vi "SIM Integrator collector (for core) (vector).vi"(8 "DNL_Simulation CallChain":string, 9 "input":dbl[](array[numeric]), 10 "width":i32, 11 "Simulation data":T1={"continuous integrator"=enum."RK 1 (Euler)", "initial time"=0.0, "final time"=0.0, "step size"=0.0, "proposed step size"=0.0, "max step size"=0.0, "min step size"=0.0, "discrete time step"=0.0, "max step ratio"=0.0, "Diag Eval Stage"=enum."Init", "Substep Index"=0, "Timestep Index"=0.0, "simulation time"=0.0, "current timestep base"=0.0, "proposed step time"=0.0, "absolute tolerance"=0.0, "relative tolerance"=0.0, "step accepted?"=FALSE, "step complete?"=FALSE, "Halt?"=FALSE, "reset integrator?"=FALSE, "machine epsilon"=0.0, "min float"=0.0, "error"={"status"=FALSE, "code"=0, "source"=""}, "Method Order"=0, "Finished Late [i-1]"=FALSE, "Discrete step?"=FALSE, "NaN and Inf check?"=FALSE, "Final Timestep Index"=0.0, "(maj+disc)or(init)?"=FALSE, "Full Solver Reset"=TRUE, "Execution Mode"=enum."Simulate to Completion", "check vector sizes?"=FALSE, "solver handles zc?"=FALSE, "Simulation Registry"={"Current Idx"=0, "Node Tags"=[], "Node Headers"=[], "Node Data"=[], "Cont State data"={"inputs"=[], "outputs"=[], "reset"=[], "lower limits"=[], "upper limits"=[], "limit types"=[], "reset types"=[], "initial conditions"=[], "reset I.C."=[], "limited?"=[], "State Names"=[]}, "DiscreteInfo"={"tick period (sec)"=0.0, "time (ticks)"=0, "fire?"=[], "registry"={"period (sec)"=[], "skew (sec)"=[], "period (tick)"=[], "skew (tick)"=[]}, "discrete \nblocks?"=FALSE, "steps per tick"=0.0, "steps to tick"=0.0, "discrete \ntick?"=FALSE}, "Disc State data"={"Disc States"=[], "State Names"=[]}, "Registry Error"={"Error Block ID"=0, "code"=0}, "ZC Indices"=[]}, "variable step solver?"=FALSE, "First Substep?"=FALSE, "Continuous States?"=FALSE} {"min float" format="%.1e"; "proposed step size" format="%.1e"; "proposed step time" format="%.1e"; "max step ratio" format="%.1e"; "min step size" format="%.1e"; "machine epsilon" format="%.1e"; "discrete time step" format="%.1e"; "max step size" format="%.1e"; "current timestep base" format="%.1e"; "final time" format="%.1e"; "simulation time" format="%.1e"; "relative tolerance" format="%.1e"; "absolute tolerance" format="%.1e"; "Substep Index" format="%.1e"; "step size" format="%.1e"; "initial time" format="%.1e"}) -> (3 "Simulation data out":T1={"continuous integrator"=enum."RK 1 (Euler)", "initial time"=0.0, "final time"=0.0, "step size"=0.0, "proposed step size"=0.0, "max step size"=0.0, "min step size"=0.0, "discrete time step"=0.0, "max step ratio"=0.0, "Diag Eval Stage"=enum."Init", "Substep Index"=0, "Timestep Index"=0.0, "simulation time"=0.0, "current timestep base"=0.0, "proposed step time"=0.0, "absolute tolerance"=0.0, "relative tolerance"=0.0, "step accepted?"=FALSE, "step complete?"=FALSE, "Halt?"=FALSE, "reset integrator?"=FALSE, "machine epsilon"=0.0, "min float"=0.0, "error"={"status"=FALSE, "code"=0, "source"=""}, "Method Order"=0, "Finished Late [i-1]"=FALSE, "Discrete step?"=FALSE, "NaN and Inf check?"=FALSE, "Final Timestep Index"=0.0, "(maj+disc)or(init)?"=FALSE, "Full Solver Reset"=TRUE, "Execution Mode"=enum."Simulate to Completion", "check vector sizes?"=FALSE, "solver handles zc?"=FALSE, "Simulation Registry"={"Current Idx"=0, "Node Tags"=[], "Node Headers"=[], "Node Data"=[], "Cont State data"={"inputs"=[], "outputs"=[], "reset"=[], "lower limits"=[], "upper limits"=[], "limit types"=[], "reset types"=[], "initial conditions"=[], "reset I.C."=[], "limited?"=[], "State Names"=[]}, "DiscreteInfo"={"tick period (sec)"=0.0, "time (ticks)"=0, "fire?"=[], "registry"={"period (sec)"=[], "skew (sec)"=[], "period (tick)"=[], "skew (tick)"=[]}, "discrete \nblocks?"=FALSE, "steps per tick"=0.0, "steps to tick"=0.0, "discrete \ntick?"=FALSE}, "Disc State data"={"Disc States"=[], "State Names"=[]}, "Registry Error"={"Error Block ID"=0, "code"=0}, "ZC Indices"=[]}, "variable step solver?"=FALSE, "First Substep?"=FALSE, "Continuous States?"=FALSE} {"min float" format="%.1e"; "proposed step size" format="%.1e"; "proposed step time" format="%.1e"; "max step ratio" format="%.1e"; "min step size" format="%.1e"; "machine epsilon" format="%.1e"; "discrete time step" format="%.1e"; "max step size" format="%.1e"; "current timestep base" format="%.1e"; "final time" format="%.1e"; "simulation time" format="%.1e"; "relative tolerance" format="%.1e"; "absolute tolerance" format="%.1e"; "Substep Index" format="%.1e"; "step size" format="%.1e"; "initial time" format="%.1e"})   [LabVIEW 2014]
uses:
  SIM simulation data.ctl
  SIM integration method.ctl
  SIM diagram eval stage.ctl
  SIMSCR Execution Mode.ctl
  SIM Simulation Registry.ctl
  SIM Registry Node Header.ctl
  SIM Registry Node Record.ctl
  SIM trigger type.ctl
  SIM solver state data.ctl
  SIM limit type.ctl
  SIM discrete data.ctl
  SIM Discrete state data.ctl
  SIM Simulation Registry Error.ctl
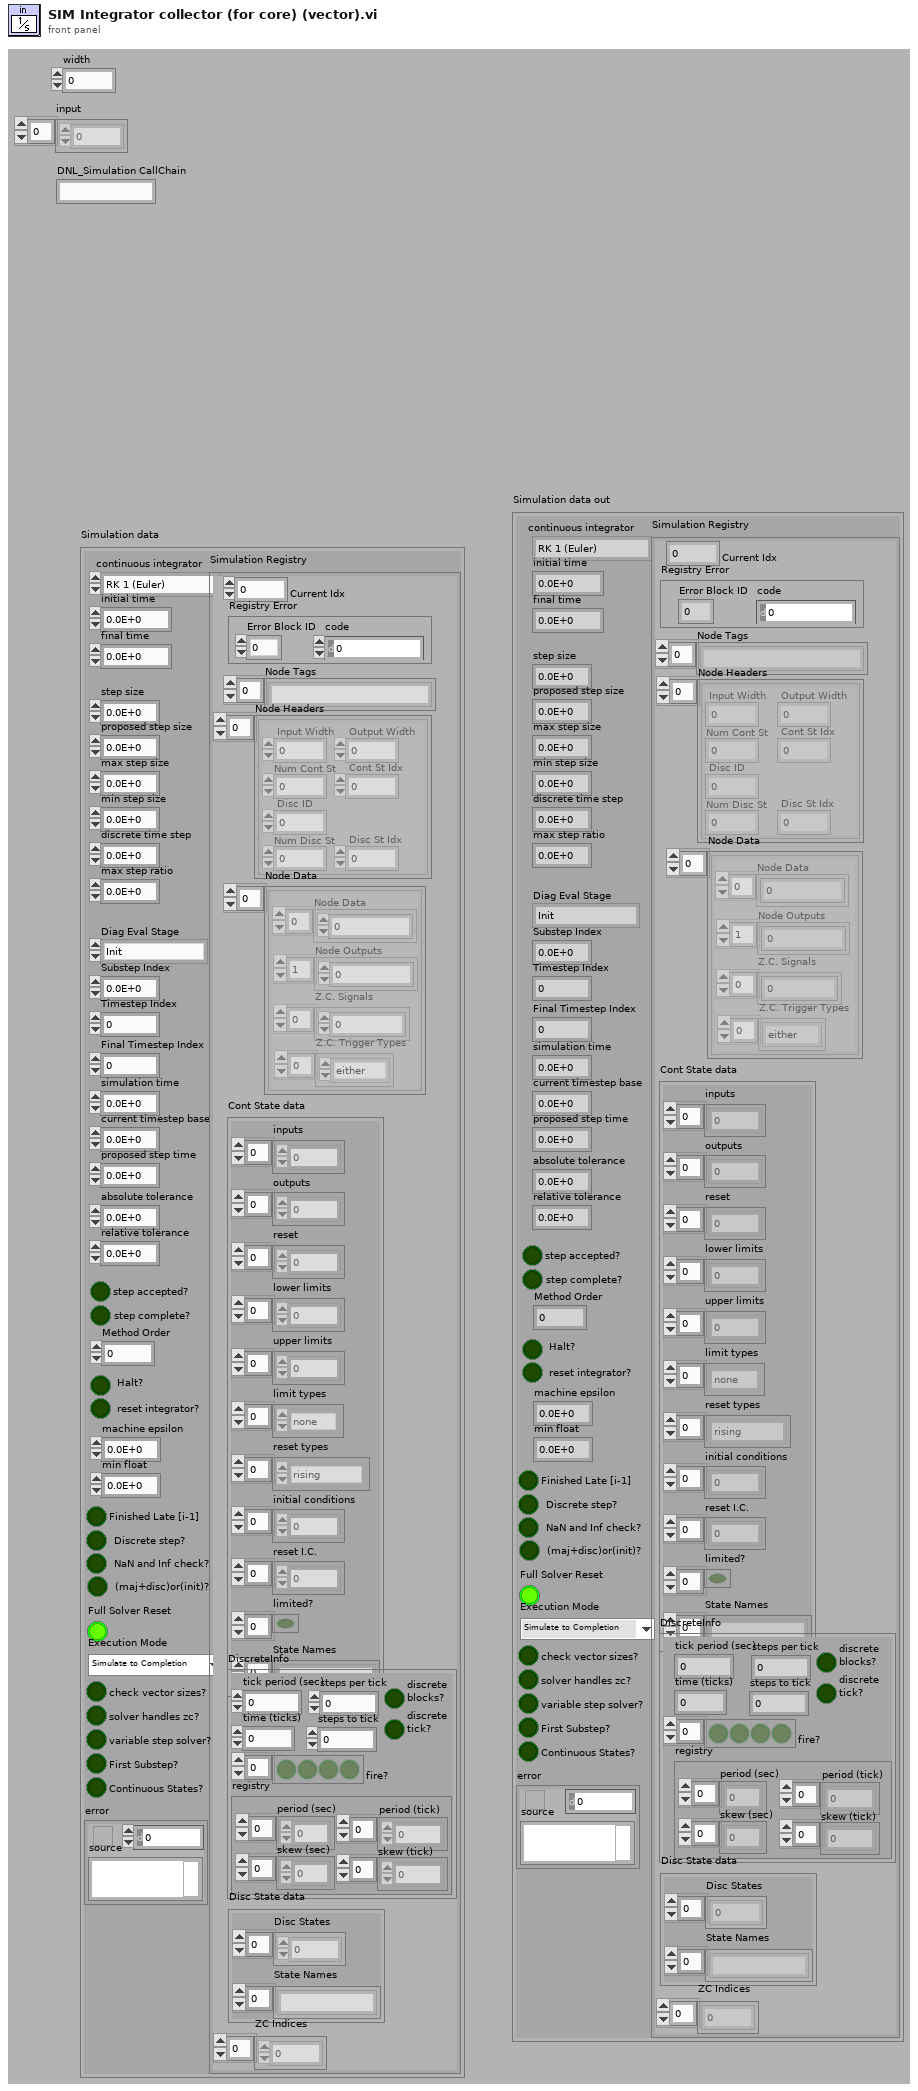
[diagram p1: front panel]
types:
  T1 = typedef "SIM simulation data.ctl" = cluster{"continuous integrator":T2, "initial time":dbl, "final time":dbl, "step size":dbl, "proposed step size":dbl, "max step size":dbl, "min step size":dbl, "discrete time step":dbl, "max step ratio":dbl, "Diag Eval Stage":T3, "Substep Index":i32, "Timestep Index":dbl, "simulation time":dbl, "current timestep base":dbl, "proposed step time":dbl, "absolute tolerance":dbl, "relative tolerance":dbl, "step accepted?":bool, "step complete?":bool, "Halt?":bool, "reset integrator?":bool, "machine epsilon":dbl, "min float":dbl, "error":errorcluster, "Method Order":u32, "Finished Late [i-1]":bool, "Discrete step?":bool, "NaN and Inf check?":bool, "Final Timestep Index":dbl, "(maj+disc)or(init)?":bool, "Full Solver Reset":bool, "Execution Mode":T4, "check vector sizes?":bool, "solver handles zc?":bool, "Simulation Registry":T5, "variable step solver?":bool, "First Substep?":bool, "Continuous States?":bool}
  T2 = typedef "SIM integration method.ctl" = enum16{"RK 1 (Euler)", "Linearizer", "State Query", "Trim Eval", "Adams", "RK 3", "RK 4", "RK 45", "BDF", "RK 2", "RK 23", "Rosenbrock", "Discrete States Only"}
  T3 = typedef "SIM diagram eval stage.ctl" = enum16{"Init", "Minor Substep", "Major Substep", "Final"}
  T4 = typedef "SIMSCR Execution Mode.ctl" = enum16{"Simulate to Completion", "Single Time-Step Simulation (Fixed Step Only)"}
  T5 = typedef "SIM Simulation Registry.ctl" = cluster{"Current Idx":i32, "Node Tags":string[], "Node Headers":T6[], "Node Data":T7[], "Cont State data":T9, "DiscreteInfo":T11, "Disc State data":T12, "Registry Error":T13, "ZC Indices":i32[]}
  T6 = typedef "SIM Registry Node Header.ctl" = cluster{"Input Width":i32, "Disc ID":i32, "Num Cont St":i32, "Cont St Idx":i32, "Num Disc St":i32, "Disc St Idx":i32, "Output Width":i32}
  T7 = typedef "SIM Registry Node Record.ctl" = cluster{"Node Data":dbl[], "Node Outputs":dbl[], "Z.C. Signals":dbl[], "Z.C. Trigger Types":T8[]}
  T8 = typedef "SIM trigger type.ctl" = enum16{"rising", "falling", "either", "none"}
  T9 = typedef "SIM solver state data.ctl" = cluster{"inputs":dbl[], "outputs":dbl[], "reset":dbl[], "lower limits":dbl[], "upper limits":dbl[], "limit types":T10[], "reset types":T8[], "initial conditions":dbl[], "reset I.C.":dbl[], "limited?":bool[], "State Names":string[]}
  T10 = typedef "SIM limit type.ctl" = enum16{"upper", "lower", "both", "none"}
  T11 = typedef "SIM discrete data.ctl" = cluster{"tick period (sec)":dbl, "time (ticks)":i32, "fire?":bool[], "registry":cluster{"period (sec)":dbl[], "skew (sec)":dbl[], "period (tick)":i32[], "skew (tick)":i32[]}, "discrete \nblocks?":bool, "steps per tick":dbl, "steps to tick":dbl, "discrete \ntick?":bool}
  T12 = typedef "SIM Discrete state data.ctl" = cluster{"Disc States":dbl[], "State Names":string[]}
  T13 = typedef "SIM Simulation Registry Error.ctl" = cluster{"Error Block ID":i32, "code":i32}
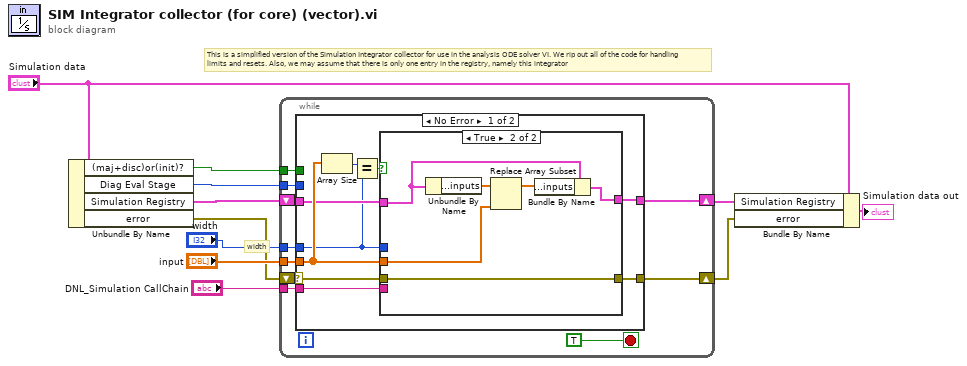
[diagram p0: block diagram]
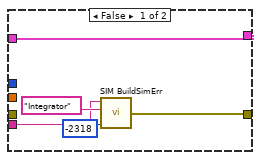
[diagram p2: hidden frame]
diagram:
  # "This is a simplified version of the Simulation Integrator collector for use in the analysis ODE solver VI. We rip out all of the code for handling\nlimits and resets. Also, we may assume that there is only one entry in the registry, namely this integrator"
  # "width"
  n1 = Unbundle By Name("Simulation data") -> ("(maj+disc)or(init)?"=w8:bool, "Diag Eval Stage"=w10:T3, "Simulation Registry"=w11:T5, "error"=w3:errorcluster)
  n2 = while {
    tunnel: w10 -> [w21]
    shift-right: [w19] -> w2
    shift-left: w3 -> [w15]
    shift-right: [w18] -> w9
    shift-left: w11 -> [w20]
    tunnel: w8 -> [w16]
    tunnel: "input" -> [w14]
    tunnel: "DNL_Simulation CallChain" -> [w13]
    tunnel: "width" -> [w12]
    stop <- TRUE stop-if-true
    n3 = case shown="No Error" w15 {
      selector: w15 -> [w28 w43]
      tunnel: w21 -> [_ _]
      tunnel: [w27 w43] -> w19
      tunnel: [w29 w42] -> w18
      tunnel: w20 -> [w23 w42]
      tunnel: w16 -> [_ _]
      tunnel: w14 -> [w30 _]
      tunnel: w13 -> [w26 _]
      tunnel: w12 -> [w22 _]
      frame No Error {
        n4 = Array Size(array=w30) -> (size(s)=w25:i32)
        n5 = Equal?(x=w25, y=w22) -> (x = y?=w24:bool)
        n6 = case shown="True" w24 {
          tunnel: w22 -> [_ _]
          tunnel: w30 -> [_ w37]
          tunnel: w23 -> [w35 w38]
          tunnel: [w35 w36] -> w29
          tunnel: w28 -> [_ w39]
          tunnel: [w32 w39] -> w27
          tunnel: w26 -> [w31 _]
          frame False {
            n7 = call "SIM BuildSimErr.vi"("error.code"=-2318, "Block Name"="Integrator" ("string"), "CallChain"=w31) -> ("Error Cluster"=w32:errorcluster)  [unwired: 1 in]
          }
          frame True {
            n8 = Unbundle By Name(w38) -> ("Cont State data.inputs"=w41:dbl[])
            n9 = Replace Array Subset(array=w41, new element=w37) -> (w40:dbl[])  [unwired: 1 in]
            n10 = Bundle By Name(cluster=w38, "Cont State data.inputs"=w40) -> (w36:T5)
          }
        }
      }
      frame Error {
      }
    }
  }
  n11 = Bundle By Name(cluster="Simulation data", "Simulation Registry"=w9, "error"=w2) -> (→"Simulation data out":T1)
